vi "HeaderAction.vi"(0 "InstrClass":refnum<class "DefaultDev.lvclass"> caption="DNL_LabVIEW Object in", 11 "error in (no error)":errorcluster caption="entrée d'erreur (pas d'erreur)") -> (4 "InstrClassOut":refnum<class "DefaultDev.lvclass"> caption="DNL_LabVIEW Object out", 6 "DataNames":string[](array[string]), 8 "Instr Name":string, 10 "HeaderString":string, 14 "DisplayNames":string[](array[string]), 15 "error out":errorcluster caption="sortie d'erreur")   [LabVIEW 2012, in "DefaultDev.lvclass"]
uses:
  DefaultDev.lvclass
  DefaultDev.lvclass/DefaultDev.ctl
  DevicesClass/BaseDevice/BaseDevice.lvclass
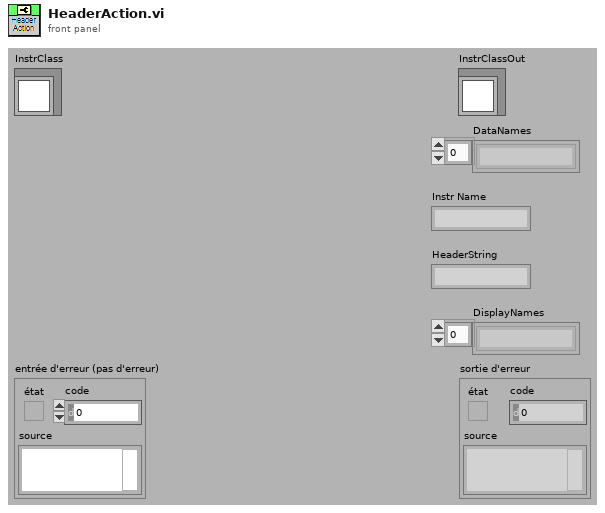
[diagram p1: front panel]
types:
  T1 = typedef "DefaultDev.lvclass/DefaultDev_Func.ctl" = enum16{"DefaultFunc (Arb)"}
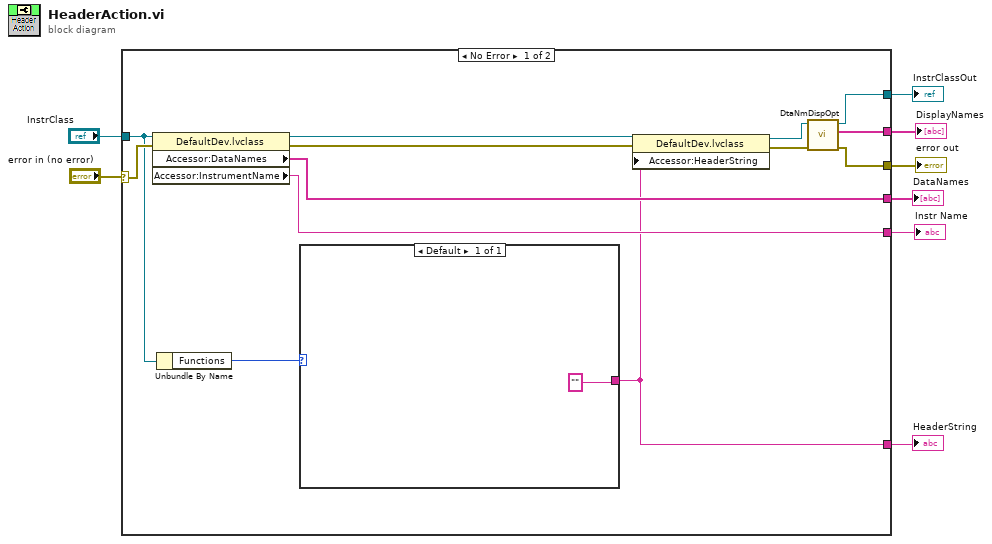
[diagram p0: block diagram]
diagram:
  n1 = case shown="No Error" "error in (no error)" {
    selector: "error in (no error)" -> [w21 w23]
    tunnel: [w14 _] -> w7
    tunnel: [w20 _] -> w6
    tunnel: "InstrClass" -> [w16 w24]
    tunnel: [w12 w23] -> w4
    tunnel: [w11 w24] -> w2
    tunnel: [w17 _] -> w3
    tunnel: [w9 _] -> w1
    frame No Error {
      n2 = property class="DefaultDev.lvclass"(reference=w16, error in=w21) -> (reference out=w19:refnum<class "DefaultDev.lvclass">, error out=w18:errorcluster, "Accessor:DataNames"=w20:string[], "Accessor:InstrumentName"=w17:string)
      n3 = Unbundle By Name(w16) -> ("Functions"=w15:T1)
      n4 = case shown="Default" w15 {
        tunnel: ["" ("HeaderString")] -> w14
        frame Default {
        }
      }
      n5 = property class="DefaultDev.lvclass"(reference=w19, error in=w18, "Accessor:HeaderString"=w14) -> (reference out=w10:refnum<class "DefaultDev.lvclass">, error out=w13:errorcluster)
      n6 = call "DtaNmDispOpt.vi"("error in (no error)"=w13, "BaseDevice en entrée"=w10) -> ("error out"=w12:errorcluster, "DisplayNames"=w9:string[], "BaseDevice en sortie"=w11:refnum<class "DefaultDev.lvclass">)  [unwired: 7 in]
    }
    frame Error {
    }
  }
  "error out" <- w4
  "InstrClassOut" <- w2
  "DataNames" <- w6
  "HeaderString" <- w7
  "Instr Name" <- w3
  "DisplayNames" <- w1
